vi "Display_Console_Thread.vi"(8 "error in (no error)":errorcluster) -> (0 "error out":errorcluster)   [LabVIEW 2020]
doc: "Display Console Process"
uses:
  controls/Event_User.ctl
  controls/Configuration_Database.ctl
  controls/Share_Data.ctl
  SubVIs/User Event - Stop/User Event - Stop.lvlib
  <vilib>/Utility/error.llb/Error Cluster From Error Code.vi
  <vilib>/ErrorRing/Error Ring.xnode
  SubVIs/Message Queue/Message Queue.lvlib
  controls/FGV_To_Do.ctl
  Controls/Display_Console.ctl
  Controls/Display_Console_local_data.ctl
  Timer/Timer.lvclass
  SubVIs/Message Queue/Enqueue Message (Single).vi
panel:
  out "Display Console":T1 {"Timing" format="%.0f seconds"}
  # "[Covers: UI1]"
  # "[Covers: UI3]"
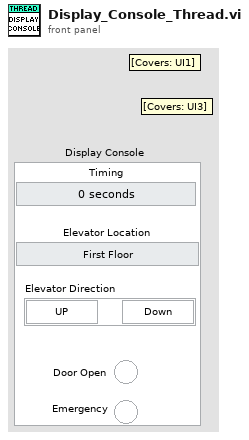
[diagram p1: front panel]
types:
  T1 = typedef "Display_Console.ctl" = cluster{"Elevator Direction":cluster{"UP":bool, "Down":bool}, "Door Open":bool, "Emergency":bool, "Elevator Location":enum16{"First Floor", "Second Floor", "Third Floor", "Fourth Floor"}, "Timing":u8}
  T2 = typedef "FGV_To_Do.ctl" = enum16{"1 - Initialize_Events", "2 - Read_Database", "3 - Initialize QMH", "Save_Database", "Read", "4 - Close_Events", "5 - Close_QMH"}
  T3 = typedef "All_Communication_Data.ctl" = cluster{"ConfigurationDatabase":T4, "QMH":T5, "User Event":T6}
  T4 = typedef "Configuration_Database.ctl" = cluster{"DoorOpen":u8, "DoorClose":u8, "TravelTime":u8, "InactivityTime":u8}
  T5 = typedef "Message Queue.lvlib/All Message Queues.ctl" = cluster{"UserConsole":refnum<queue>, "DisplayConsole":refnum<queue>, "SensorInterface":refnum<queue>}
  T6 = typedef "Event_User.ctl" = cluster{"User Event - Stop":refnum<user-event>, "User Event - Error":refnum<user-event>}
  T7 = typedef "Display_Console_local_data.ctl" = cluster{"data":T8, "Display Console":T1}
  T8 = typedef "Share_Data.ctl" = cluster{"ConfigurationDatabase":T4, "User Event":T6}
  T9 = enum16{"First Floor", "Second Floor", "Third Floor", "Fourth Floor"}
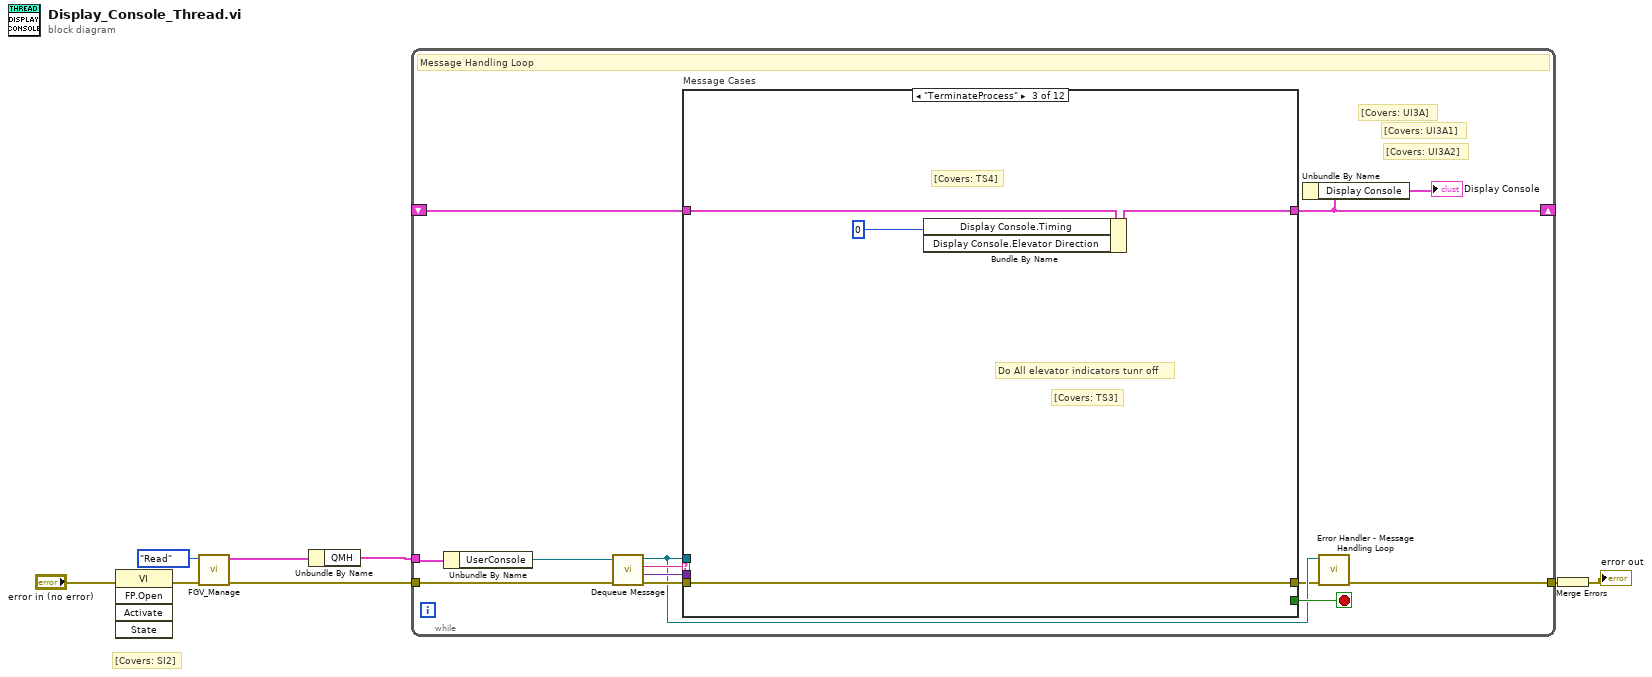
[diagram p0: block diagram]
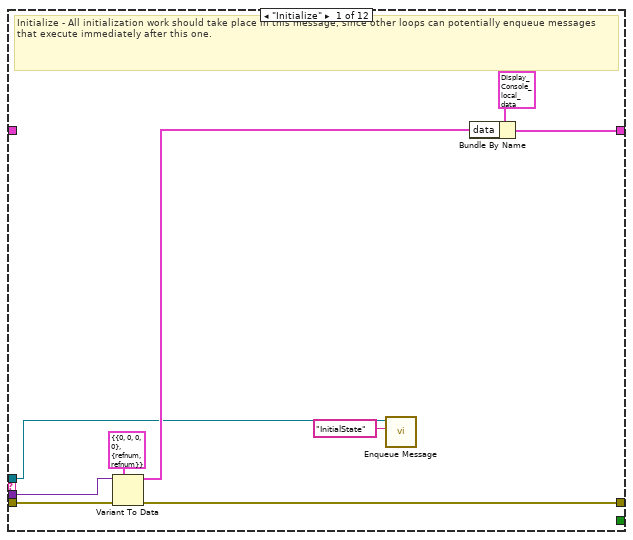
[diagram p2: hidden frame]
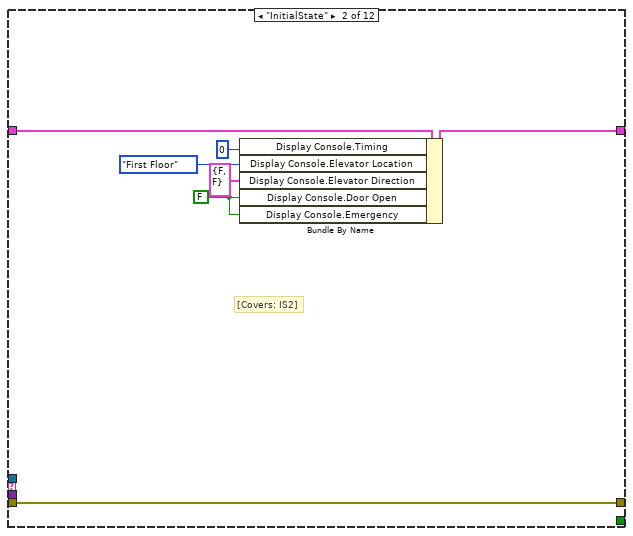
[diagram p3: hidden frame]
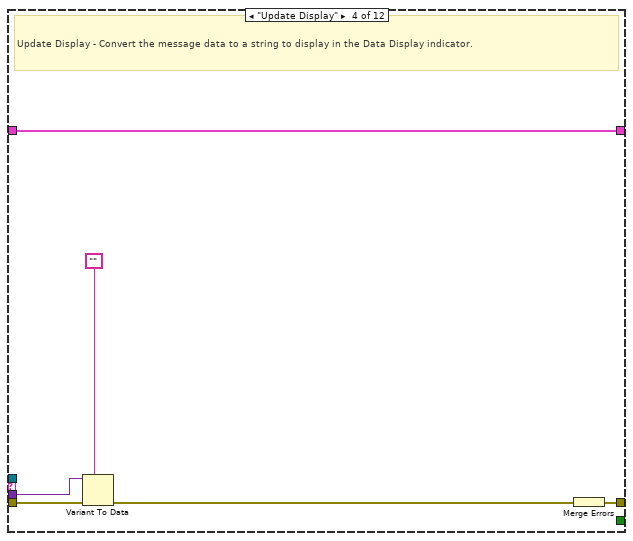
[diagram p4: hidden frame]
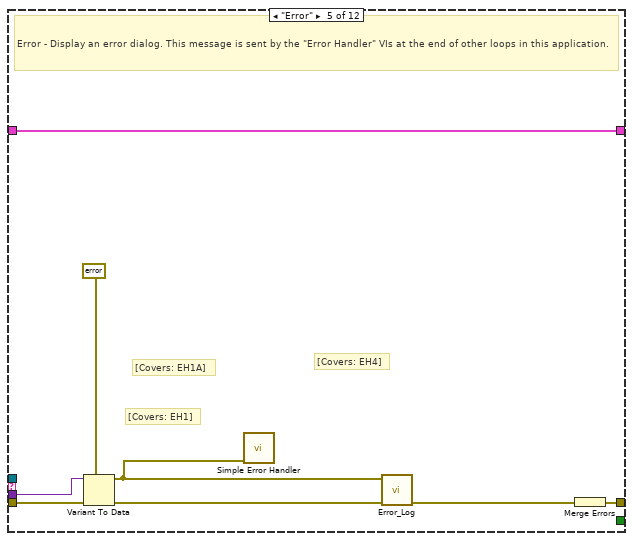
[diagram p5: hidden frame]
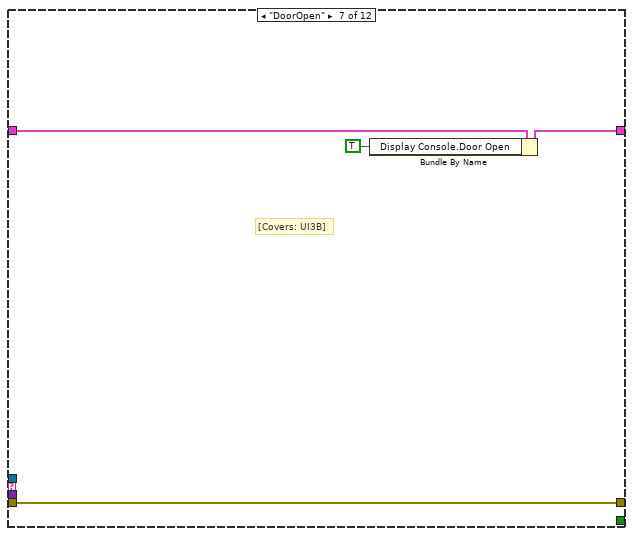
[diagram p7: hidden frame]
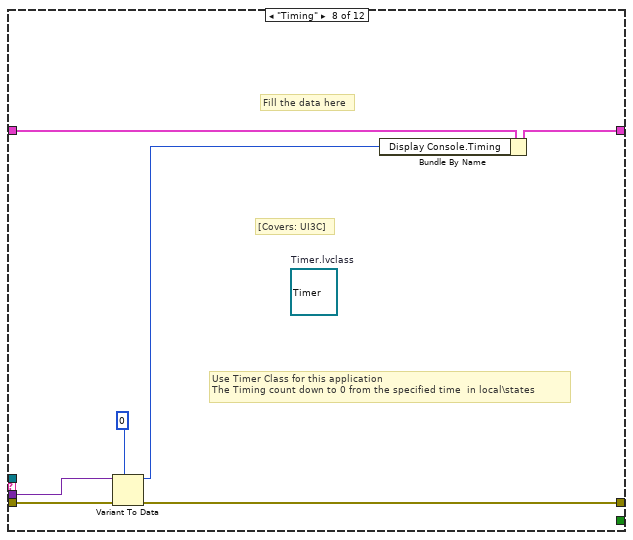
[diagram p8: hidden frame]
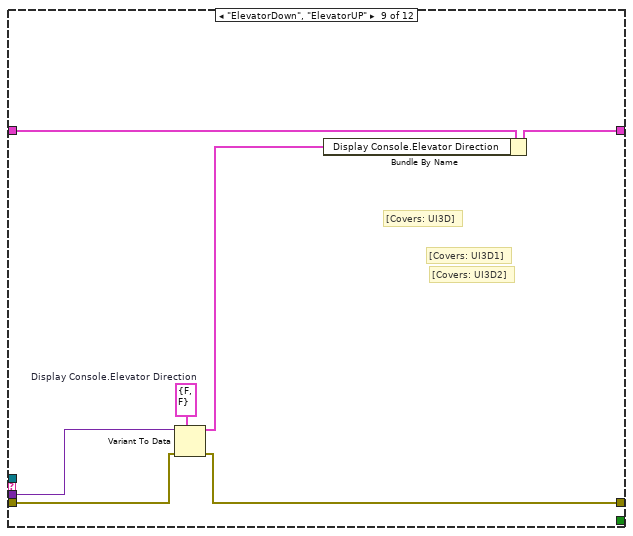
[diagram p9: hidden frame]
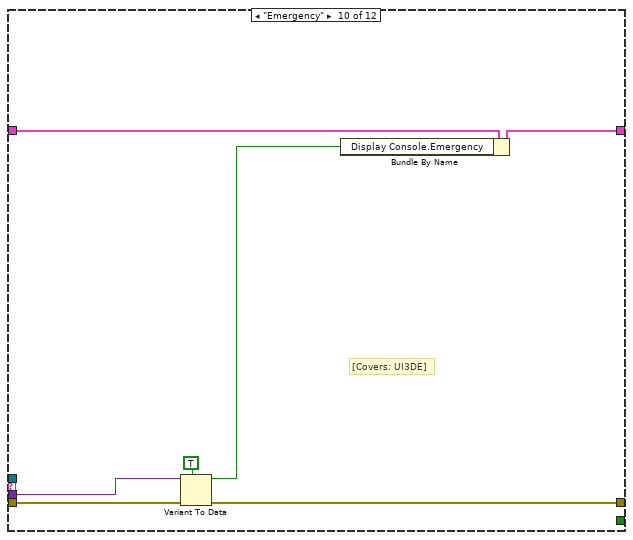
[diagram p10: hidden frame]
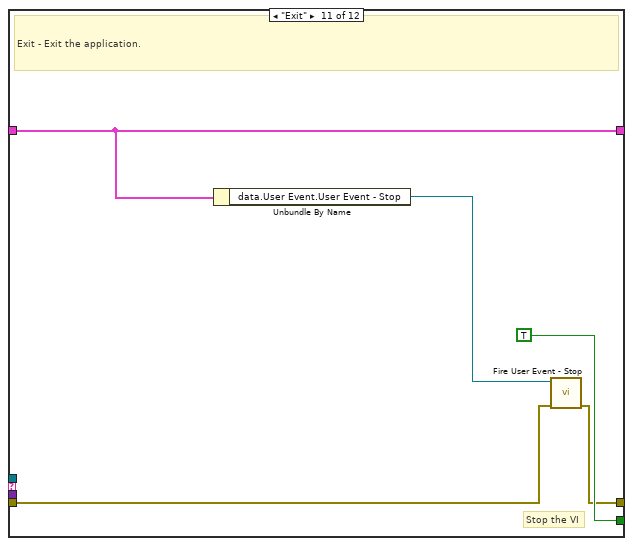
[diagram p11: hidden frame]
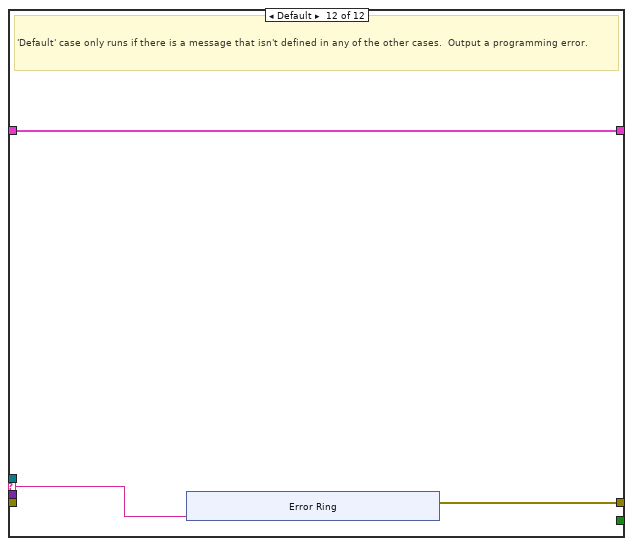
[diagram p12: hidden frame]
diagram:
  # "[Covers: SI2]"
  n1 = invoke class="VI" method="FP.Open"(error in="error in (no error)") -> (error out=w1:errorcluster)  [unwired: 4 in, 4 out]
  n2 = call "FGV_Manage.vi"("error in (no error)"=w1, "To do"=FGV_To_Do."Read") -> ("error out"=w3:errorcluster, "All_Communication OUT"=w6:T3)  [unwired: 8 in]
  n3 = Unbundle By Name(w6) -> ("QMH"=w7:T5)
  n4 = while {
    tunnel: w7 -> [w12]
    shift-right: [w10] -> _
    shift-left: _ -> [w21]
    tunnel: w3 -> [w19]
    tunnel: [w14] -> w4
    stop <- w20 stop-if-true
    # "[Covers: UI3A2]"
    # "[Covers: UI3A1]"
    # "[Covers: UI3A]"
    # "Message Handling Loop"
    n5 = Unbundle By Name(w12) -> ("UserConsole"=w11:refnum<queue>)
    n6 = call "Dequeue Message.vi"("error in (no error)"=w19, "Message Queue"=w11) -> ("error out"=w18:errorcluster, "Message Data"=w16:variant, "Message"=w17:string, "dup Message Queue"=w15:refnum<queue>)  [unwired: 6 in]
    n7 = case "Message Cases" shown="\"TerminateProcess\"" w17 {
      selector: w17 -> [_ _ _ _ _ _ _ _ _ _ _ w88]
      tunnel: w15 -> [w22 _ _ _ _ _ _ _ _ _ _ _]
      tunnel: w18 -> [w29 w37 w41 w45 w55 w57 w61 w66 w73 w80 w84 _]
      tunnel: [w27 w37 w41 w46 w51 w57 w61 w63 w69 w76 w83 w89] -> w13
      tunnel: w21 -> [_ w36 w40 w47 w54 w56 w60 w68 w75 w82 w86 w90]
      tunnel: [w25 w35 w39 w47 w54 w56 w59 w67 w74 w81 w86 w90] -> w10
      tunnel: [_ _ _ _ _ _ _ _ _ _ TRUE _] -> w20
      tunnel: w16 -> [w28 _ _ w44 w53 _ _ w65 w71 w79 _ _]
      frame "Initialize" {
        # "Initialize - All initialization work should take place in this message, since other loops can potentially enqueue messages that execute immediately after this one."
        n8 = Variant To Data(error in=w29, type=T8 {"ConfigurationDatabase"={"DoorOpen"=0, "DoorClose"=0, "TravelTime"=0, "InactivityTime"=0}, "User Event"={"User Event - Stop"=refnum, "User Event - Error"=refnum}} ("Share_Data"), Variant=w28) -> (data=w26:T8, error out=w27:errorcluster)
        n9 = call-poly "Enqueue Message.vi"("Message"="InitialState", "Message Queue"=w22) -> ()  [unwired: 8 in, 2 out]
        n10 = Bundle By Name(cluster=T7 {"data"={"ConfigurationDatabase"={"DoorOpen"=0, "DoorClose"=0, "TravelTime"=0, "InactivityTime"=0}, "User Event"={"User Event - Stop"=refnum, "User Event - Error"=refnum}}, "Display Console"={"Elevator Direction"={"UP"=FALSE, "Down"=FALSE}, "Door Open"=FALSE, "Emergency"=FALSE, "Elevator Location"=enum."First Floor", "Timing"=0}} ("Cluster"), "data"=w26) -> (w25:T7)
      }
      frame "InitialState" {
        w31 = FALSE ("Display Console.Door Open")
        # "[Covers: IS2]"
        n11 = Bundle By Name(cluster=w36, "Display Console.Timing"=u8 0, "Display Console.Elevator Location"=T9."First Floor", "Display Console.Elevator Direction"=cluster{"UP":bool, "Down":bool} {"UP"=FALSE, "Down"=FALSE}, "Display Console.Door Open"=w31, "Display Console.Emergency"=w31) -> (w35:T7)
      }
      frame "TerminateProcess" {
        # "[Covers: TS3]"
        # "Do All elevator indicators tunr off"
        # "[Covers: TS4]"
        n12 = Bundle By Name(cluster=w40, "Display Console.Timing"=u8 0) -> (w39:T7)  [unwired: 1 in]
      }
      frame "Update Display" {
        # "Update Display - Convert the message data to a string to display in the Data Display indicator."
        n13 = Variant To Data(error in=w45, type="", Variant=w44) -> (error out=w42:errorcluster)  [unwired: 1 out]
        n14 = Merge Errors(w42) -> (w46:errorcluster)
      }
      frame "Error" {
        # "[Covers: EH1A]"
        # "[Covers: EH4]"
        # "[Covers: EH1]"
        # "Error - Display an error dialog. This message is sent by the \"Error Handler\" VIs at the end of other loops in this application."
        n15 = Variant To Data(error in=w55, type=errorcluster {"status"=FALSE, "code"=0, "source"=""} ("error constant"), Variant=w53) -> (data=w49:errorcluster, error out=w50:errorcluster)
        n16 = call <vilib>:"Simple Error Handler.vi"("error in (no error)"=w49) -> ()  [unwired: 4 in, 5 out]
        n17 = call "Error_Log.vi"("error in"=w50, "Error report"=w49) -> ("error out"=w48:errorcluster)  [unwired: 9 in]
        n18 = Merge Errors(w48) -> (w51:errorcluster)
      }
      frame "Idle" {
      }
      frame "DoorOpen" {
        # "[Covers: UI3B]"
        n19 = Bundle By Name(cluster=w60, "Display Console.Door Open"=TRUE) -> (w59:T7)
      }
      frame "Timing" {
        (unwired) refnum<class "Timer.lvclass"> refnum  # Timer.lvclass
        # "Fill the data here"
        # "Use Timer Class for this application\nThe Timing count down to 0 from the specified time  in local\\states"
        # "[Covers: UI3C]"
        n20 = Variant To Data(error in=w66, type=u8 0 ("Display Console.Timing"), Variant=w65) -> (data=w62:u8, error out=w63:errorcluster)
        n21 = Bundle By Name(cluster=w68, "Display Console.Timing"=w62) -> (w67:T7)
      }
      frame "ElevatorDown", "ElevatorUP" {
        w72 = cluster{"UP":bool, "Down":bool} {"UP"=FALSE, "Down"=FALSE}  # Display Console.Elevator Direction
        # "[Covers: UI3D1]"
        # "[Covers: UI3D2]"
        # "[Covers: UI3D]"
        n22 = Variant To Data(error in=w73, type=w72, Variant=w71) -> (data=w70:cluster{"UP":bool, "Down":bool}, error out=w69:errorcluster)
        n23 = Bundle By Name(cluster=w75, "Display Console.Elevator Direction"=w70) -> (w74:T7)
      }
      frame "Emergency" {
        # "[Covers: UI3DE]"
        n24 = Variant To Data(error in=w80, type=TRUE ("Display Console.Elevator Direction.UP"), Variant=w79) -> (data=w77:bool, error out=w76:errorcluster)
        n25 = Bundle By Name(cluster=w82, "Display Console.Emergency"=w77) -> (w81:T7)
      }
      frame "Exit" {
        # "Stop the VI"
        # "Exit - Exit the application."
        n26 = Unbundle By Name(w86) -> ("data.User Event.User Event - Stop"=w85:refnum<user-event>)
        n27 = call "Fire User Event - Stop.vi"("error in (no error)"=w84, "User Event - Stop"=w85) -> ("error out"=w83:errorcluster)  [unwired: 9 in]
      }
      frame Default {
        # "'Default' case only runs if there is a message that isn't defined in any of the other cases.  Output a programming error."
        n28 = xnode "Error Ring"("parameter 0"=w88) -> ("error out"=w89:errorcluster)
      }
    }
    n29 = Unbundle By Name(w10) -> ("Display Console"=→"Display Console":T1)
    n30 = call "Error Handler - Message Handling Loop.vi"("error in (no error)"=w13, "Message Queue"=w15) -> ("dup error in"=w14:errorcluster)  [unwired: 8 in, 1 out]
  }
  n31 = Merge Errors(w4) -> (→"error out":errorcluster)
